vi "AxisCutter(Arduino).vi"(0 "수신":string) -> (7 "Axis":string, 13 "END":string, 14 "L":i32, 15 "R":i32, 16 "M":i32, 17 "A":i32, 18 "B":i32, 19 "C":i32)   [LabVIEW 2013]
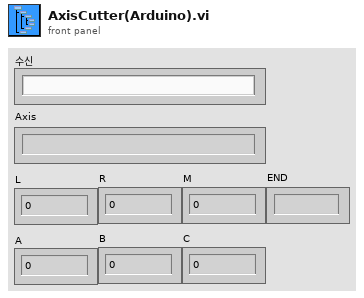
[diagram p1: front panel]
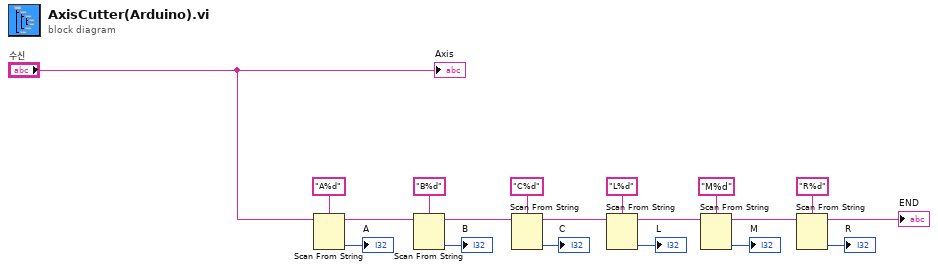
[diagram p0: block diagram]
diagram:
  n1 = Scan From String(format string="A%d" ("포맷 문자열"), input string="수신") -> (remaining string=w7:string, output 1=→"A":i32)  [unwired: 3 in, 2 out]
  n2 = Scan From String(format string="B%d" ("포맷 문자열"), input string=w7) -> (remaining string=w6:string, output 1=→"B":i32)  [unwired: 3 in, 2 out]
  n3 = Scan From String(format string="C%d" ("포맷 문자열"), input string=w6) -> (remaining string=w5:string, output 1=→"C":i32)  [unwired: 3 in, 2 out]
  n4 = Scan From String(format string="L%d" ("포맷 문자열"), input string=w5) -> (remaining string=w3:string, output 1=→"L":i32)  [unwired: 3 in, 2 out]
  n5 = Scan From String(format string="M%d" ("포맷 문자열"), input string=w3) -> (remaining string=w2:string, output 1=→"M":i32)  [unwired: 3 in, 2 out]
  n6 = Scan From String(format string="R%d" ("포맷 문자열"), input string=w2) -> (remaining string=→"END":string, output 1=→"R":i32)  [unwired: 3 in, 2 out]
  "Axis" <- "수신"
